vi "average.vi"() -> ()   [LabVIEW 2012]
panel:
  out "x/y":dbl
  in  "Numeric 3":dbl
  in  "Numeric 2":dbl
  in  "Numeric":dbl
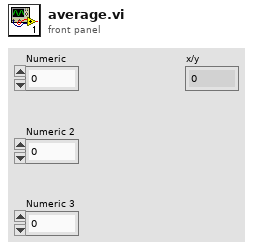
[diagram p1: front panel]
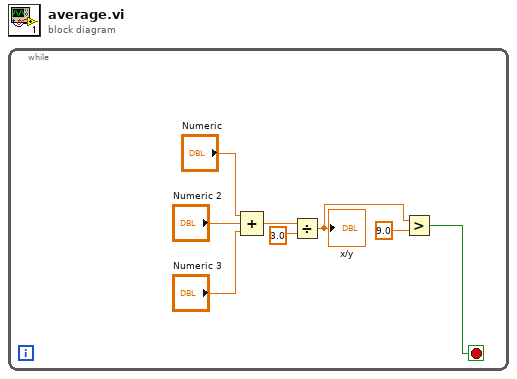
[diagram p0: block diagram]
diagram:
  n1 = while {
    stop <- w1 stop-if-true
    n2 = Compound Arithmetic op=ADD("Numeric", "Numeric 2", "Numeric 3") -> (w4:dbl)
    n3 = Divide(x=w4, y=3.0) -> (x/y=w3:dbl)
    "x/y" <- w3
    n4 = Greater?(x=w3, y=9.0) -> (0:w1:bool)
  }
